vi "Read COM port.vi"(8 "error in (no error)":errorcluster, 11 "COM Port D Element in":refnum<class "COM Port D Element.lvclass">) -> (0 "error out":errorcluster, 2 "COM port":refnum<visa-resource-name>, 3 "COM Port D Element out":refnum<class "COM Port D Element.lvclass">)   [LabVIEW 2018, in "D Datagrid Library.lvlib" / "COM Port D Element.lvclass"]
uses:
  COM Port D Element.lvclass
  C:/dev/D Datagrid/String Dropdown D Element/String dropdown D Element.lvclass
  String Dropdown D Element/String dropdown D Element.lvclass/String dropdown D Element.ctl
  String Dropdown D Element/Read Strings.vi
  String Dropdown D Element/Read value.vi
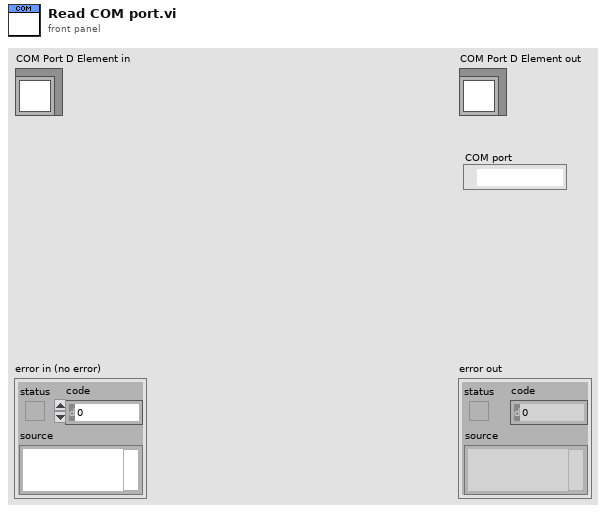
[diagram p1: front panel]
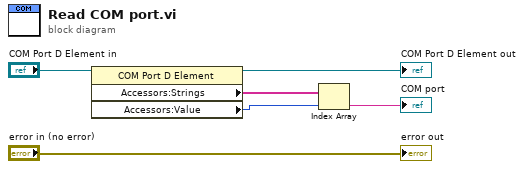
[diagram p0: block diagram]
diagram:
  n1 = property class="COM Port D Element"(reference="COM Port D Element in") -> (reference out=→"COM Port D Element out":refnum<class "COM Port D Element.lvclass">, "Accessors:Strings"=w2:string[], "Accessors:Value"=w3:i32)  [unwired: 1 in, 1 out]
  n2 = Index Array(array=w2, index=w3) -> (element=→"COM port":string)
  "error out" <- "error in (no error)"
